vi "Swerve Drive Visuals.vi"(9 "Steer Angles (degrees)":T1, 10 "Drive Velocities (ft/s)":T1, 11 "Pod Setpoints (ft/s and deg)":T2) -> (2 "Swerve Visualizer":cluster{dbl[], dbl[]}[](graph), 3 "Pod Comparisons (Diff -> Setpoint - Actual)":T3)   [LabVIEW 2025]
uses:
  swerve-template/Type Definitions/Data/Pod Setpoints.ctl
  <vilib>/Analysis/coordinate.llb/Angle Range (Degree).ctl
  <vilib>/Analysis/coordinate.llb/Angle Units.ctl
  <vilib>/Analysis/coordinate.llb/Wrap Angle (array).vi
  <vilib>/Analysis/NI_AAL_Angle.lvlib
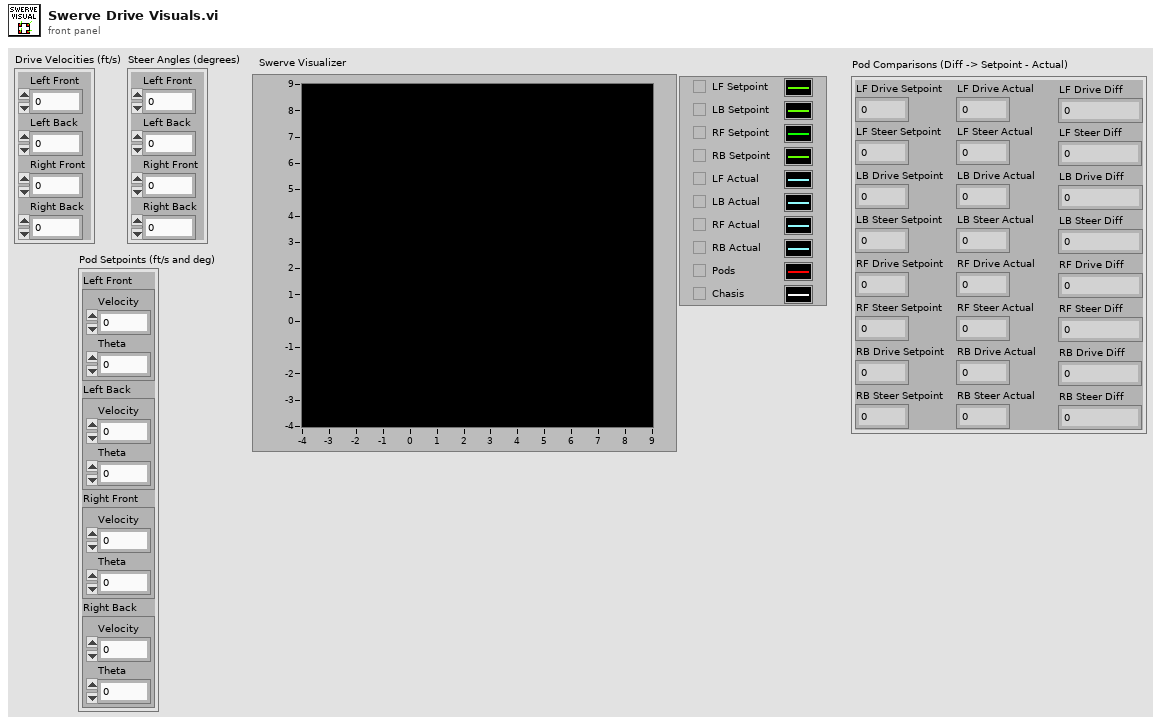
[diagram p1: front panel]
types:
  T1 = cluster{"Left Front":dbl, "Left Back":dbl, "Right Front":dbl, "Right Back":dbl}
  T2 = typedef "Pod Setpoints.ctl" = cluster{"Left Front":cluster{"Velocity":dbl, "Theta":dbl}, "Left Back":cluster{"Velocity":dbl, "Theta":dbl}, "Right Front":cluster{"Velocity":dbl, "Theta":dbl}, "Right Back":cluster{"Velocity":dbl, "Theta":dbl}}
  T3 = cluster{"LF Drive Setpoint":dbl, "LF Steer Setpoint":dbl, "LB Drive Setpoint":dbl, "LB Steer Setpoint":dbl, "RF Drive Setpoint":dbl, "RF Steer Setpoint":dbl, "RB Drive Setpoint":dbl, "RB Steer Setpoint":dbl, "LF Drive Actual":dbl, "LF Steer Actual":dbl, "LB Drive Actual":dbl, "LB Steer Actual":dbl, "RF Drive Actual":dbl, "RF Steer Actual":dbl, "RB Drive Actual":dbl, "RB Steer Actual":dbl, "LF Drive Diff":dbl, "LF Steer Diff":dbl, "LB Drive Diff":dbl, "LB Steer Diff":dbl, "RF Drive Diff":dbl, "RF Steer Diff":dbl, "RB Drive Diff":dbl, "RB Steer Diff":dbl}
  T4 = typedef "NI_AAL_Angle.lvlib/Angle Units.ctl" = i32
  T5 = typedef "NI_AAL_Angle.lvlib/Angle Range (Degree).ctl" = u16
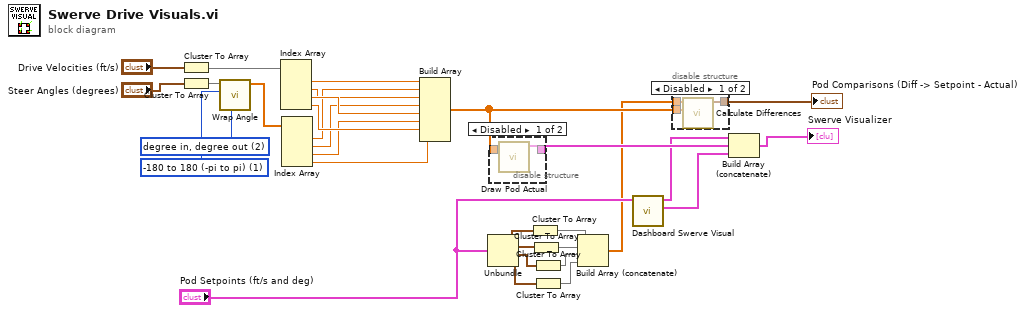
[diagram p0: block diagram]
diagram:
  w23 = T4 2 items=["radian in, radian out", "radian in, degree out", "degree in, degree out", "degree in, radian out"] ("angle units")
  w22 = T5 1 items=["none", "-180 to 180 (-pi to pi)", "0 to 360 (0 to 2pi)"] ("angle range")
  n1 = Cluster To Array(cluster="Drive Velocities (ft/s)") -> (array=w11:dbl[])
  n2 = Cluster To Array(cluster="Steer Angles (degrees)") -> (array=w20:dbl[])
  n3 = call-poly <vilib>:"Wrap Angle.vi"("angle units"=w23, "angle range"=w22, "Angle In"=w20) -> ("Angle Out"=w21:dbl[])  [unwired: 7 in, 1 out]
  n4 = Index Array(array=w11) -> (element #1=w12:dbl, element #2=w14:dbl, element #3=w16:dbl, element #4=w18:dbl)  [unwired: 4 in]
  n5 = Index Array(array=w21) -> (element #1=w13:dbl, element #2=w15:dbl, element #3=w17:dbl, element #4=w19:dbl)  [unwired: 4 in]
  n6 = Build Array(w12, w13, w14, w15, w16, w17, w18, w19) -> (w25:dbl[])
  n7 = Unbundle("Pod Setpoints (ft/s and deg)") -> ("Left Front"=w3:cluster{"Velocity":dbl, "Theta":dbl}, "Left Back"=w4:cluster{"Velocity":dbl, "Theta":dbl}, "Right Front"=w5:cluster{"Velocity":dbl, "Theta":dbl}, "Right Back"=w6:cluster{"Velocity":dbl, "Theta":dbl})
  n8 = disable-structure shown="Disabled" {
    disable-tunnel: [w33 _] -> w28
    disable-tunnel: w25 -> [w32 _]
    frame Disabled {
      n9 = call "Draw Pod Actual.vi"("Pod Sensor Readings"=w32) -> ("Actual Pod Vectors"=w33:cluster{dbl[], dbl[]}[])  [unwired: 10 in]
    }
    frame Enabled {
    }
  }
  n10 = Cluster To Array(cluster=w3) -> (array=w7:dbl[])
  n11 = Cluster To Array(cluster=w4) -> (array=w8:dbl[])
  n12 = Cluster To Array(cluster=w5) -> (array=w9:dbl[])
  n13 = Cluster To Array(cluster=w6) -> (array=w10:dbl[])
  n14 = Build Array (concatenate)(w7, w8, w9, w10) -> (w24:dbl[])
  n15 = call "Dashboard Swerve Visual.vi"("Pod Setpoints (ft/s and deg)"="Pod Setpoints (ft/s and deg)") -> ("Robot"=w29:cluster{dbl[], dbl[]}[], "Pod Vectors"=w27:cluster{dbl[], dbl[]}[])  [unwired: 9 in]
  n16 = disable-structure shown="Disabled" {
    disable-tunnel: [w36 _] -> w26
    disable-tunnel: w25 -> [w35 _]
    disable-tunnel: w24 -> [w34 _]
    frame Disabled {
      n17 = call "Calculate Differences.vi"("Actual"=w35, "Setpoint"=w34) -> ("Pod Comparisons (Diff -> Setpoint - Actual)"=w36:T3)  [unwired: 9 in]
    }
    frame Enabled {
    }
  }
  "Pod Comparisons (Diff -> Setpoint - Actual)" <- w26
  n18 = Build Array (concatenate)(w27, w28, w29) -> (→"Swerve Visualizer":cluster{dbl[], dbl[]}[])
